vi "EPOS2N~1.VI"() -> ()   [LabVIEW 2017]
doc: "Example of controlling 1 EPOS2 drive in current mode."
uses:
  <vilib>/addons/Maxon Motor/EPOS2 CANopen/EPOS2 Support Files/Typedefs/EPOS2 Status Word PVM.ctl
  <vilib>/addons/Maxon Motor/EPOS2 CANopen/EPOS2 Support Files/Typedefs/EPOS2 Data Output Current.ctl
  <vilib>/addons/Maxon Motor/EPOS2 CANopen/EPOS2 Support Files/Typedefs/EPOS2 Control Word PVM.ctl
  <vilib>/addons/Maxon Motor/EPOS2 CANopen/EPOS2 Support Files/Typedefs/EPOS2 Config Data Input Current.ctl
  <vilib>/addons/Maxon Motor/EPOS2 CANopen/EPOS2 Support Files/Typedefs/EPOS2 Velocity Units.ctl
  <vilib>/Platform/TimedLoop/XDataNode/timing_clust.ctl
  <vilib>/Platform/TimedLoop/XDataNode/nitl_modes.ctl
  <vilib>/Platform/TimedLoop/XDataNode/wakeup.ctl
  <vilib>/addons/Maxon Motor/EPOS2 CANopen/EPOS2 Support Files/Polymorphic SubVIs/Config/EPOS2 Current Mode Configure.vi
  <vilib>/addons/Maxon Motor/EPOS2 CANopen/EPOS2 Support Files/Polymorphic SubVIs/Write PDO/EPOS2 Current Mode Write.vi
  <vilib>/addons/Maxon Motor/EPOS2 CANopen/EPOS2 Support Files/Polymorphic SubVIs/Read PDO/EPOS2 Current Mode Read.vi
  <vilib>/addons/Maxon Motor/EPOS2 CANopen/CANopen/sbCANopenBaseClass.lvclass
  <vilib>/Platform/TimedLoop/XDataNode/XDataNode.xnode
  <vilib>/Platform/TimedLoop/XDataNode/XDNodeRunTimeDep.lvlib
  <vilib>/addons/Maxon Motor/EPOS2 CANopen/EPOS2 Library.lvlib
  <vilib>/addons/Maxon Motor/EPOS2 CANopen/CANopen/CANopen IndCom Interface/sdCANopenIndCom.lvclass
panel:
  in  "Node ID 2":u8=1
  out "error out 2":errorcluster
  in  "stop 2":bool
  out "Status 2":T1
  in  "Current 2":i32(slide) scale=-1000.0..1000.0
  in  "Enable 2":bool
  out "Data Output 2":T2
  out "Data Output":T2
  in  "Enable":bool
  in  "Current":i32(slide) scale=-1000.0..1000.0
  in  "Node ID":u8=1
  out "error out":errorcluster
  out "Status":T1
  in  "stop":bool
  # "This Example VI demonstrates how to control the current of an EPOS2 drive using a CANopen interface.\n\nThis VI must be run from a LabVIEW Project. An Example Projects can be found at: \nC:\\Program Files\\National Instruments\\LabVIEW 2015\\examples\\Maxon Motor\\Maxon EPOS2\nor simliar relative path to current LabVIEW version install location for all opperating systems"
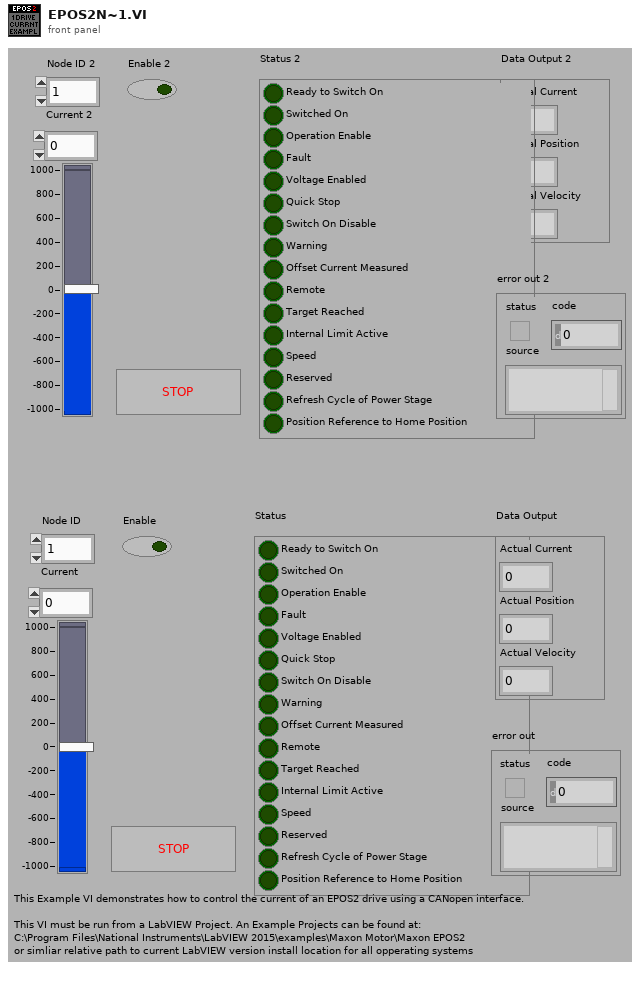
[diagram p1: front panel]
types:
  T1 = typedef "EPOS2 Library.lvlib/EPOS2 Status Word PVM.ctl" = cluster{"Ready to Switch On":bool, "Switched On":bool, "Operation Enable":bool, "Fault":bool, "Voltage Enabled":bool, "Quick Stop":bool, "Switch On Disable":bool, "Warning":bool, "Offset Current Measured":bool, "Remote":bool, "Target Reached":bool, "Internal Limit Active":bool, "Speed":bool, "Reserved":bool, "Refresh Cycle of Power Stage":bool, "Position Reference to Home Position":bool}
  T2 = typedef "EPOS2 Library.lvlib/EPOS2 Data Output Current.ctl" = cluster{"Actual Current":i16, "Actual Position":i32, "Actual Velocity":i32}
  T3 = typedef "EPOS2 Library.lvlib/EPOS2 Config Data Input Current.ctl" = cluster{"Velocity Units":T4, "Max Velocity":i32}
  T4 = typedef "EPOS2 Library.lvlib/EPOS2 Velocity Units.ctl" = i8
  T5 = typedef "EPOS2 Library.lvlib/EPOS2 Control Word PVM.ctl" = cluster{"Switch On":bool, "Enable Voltage":bool, "Quick Stop":bool, "Enable Operation":bool, "Reserved 0":bool, "Reserved 1":bool, "Reserved 2":bool, "Fault Reset":bool, "Halt":bool}
  T6 = typedef "XDNodeRunTimeDep.lvlib/timing_clust.ctl" = cluster{"Expected End [f-1]":u64, "Actual End [f-1]":u64, "Finished Late? [f-1]":bool, "Expected End [i-1]":u64, "Actual End [i-1]":u64, "Finished Late? [i-1]":bool, "Expected Start [i]":u64, "Actual Start [i]":u64, "Expected Start [f]":u64, "Actual Start [f]":u64, "Source Name":string, "Structure Name":string, "Period":i64, "Deadline":i64, "Offset":i64, "Start":i64, "Priority":i32, "Timeout":i32, "Mode":T7, "Wakeup Reason":T8, "Error":errorcluster, "Source Type":string, "Secondary Source Type":string, "Global End Time":u64, "Global Start Time":u64, "Frame Duration":u64, "Iteration Duration":u64, "Assigned CPU":i32, "I/O Scan Engine Mode":u32}
  T7 = typedef "XDNodeRunTimeDep.lvlib/nitl_modes.ctl" = enum32{"No Change", "Process missed periods, maintain original phase", "Discard missed periods, maintain original phase", "Process missed periods, ignore original phase", "Discard missed periods, ignore original phase"}
  T8 = typedef "XDNodeRunTimeDep.lvlib/wakeup.ctl" = enum32{"Normal", "Aborted", "Asynchronous wakeup", "Timing source error", "Timed loop error", "Timeout"}
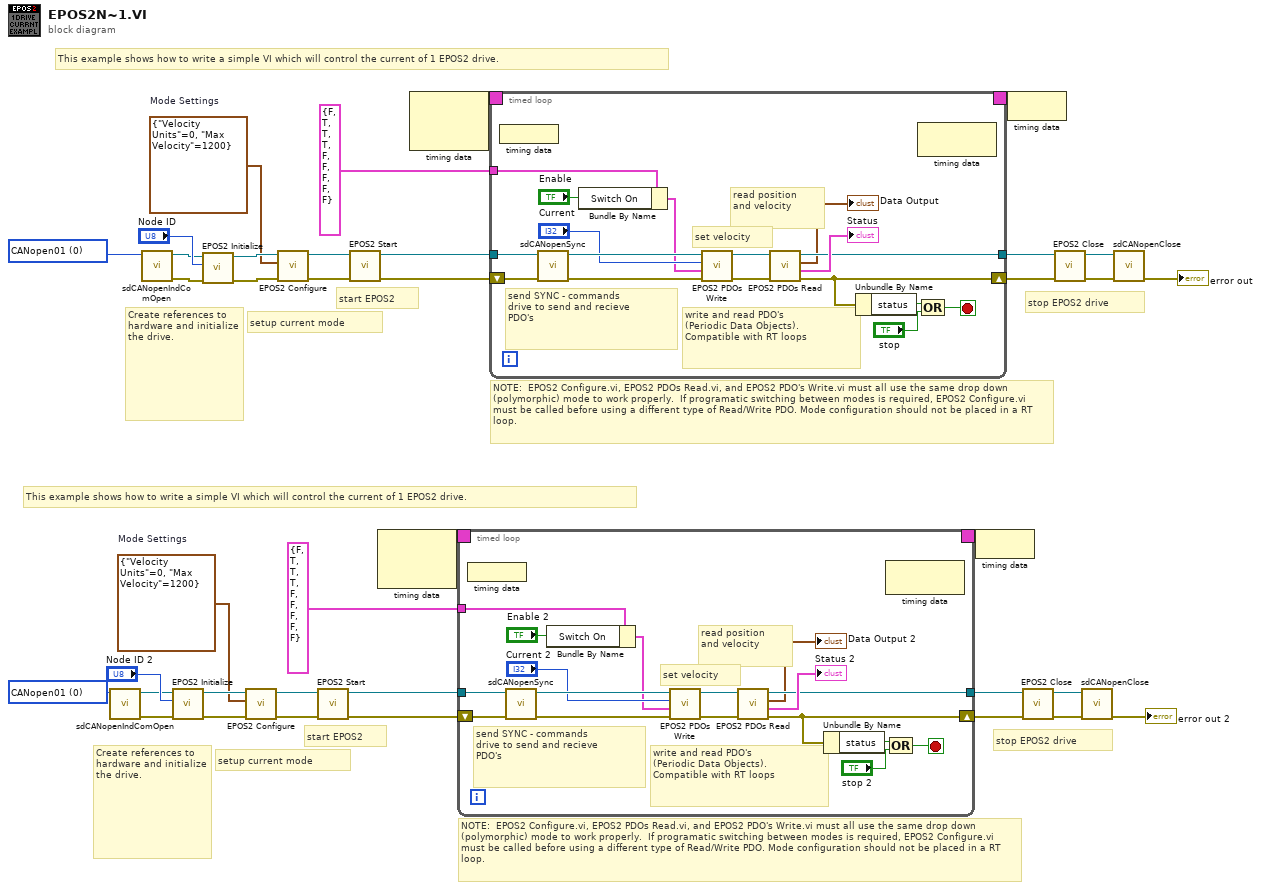
[diagram p0: block diagram]
diagram:
  w2 = u32 0 items=["CANopen01", "CANopen02", "CANopen03", "CANopen04", "CANopen05", "CANopen06", "CANopen07", "CANopen08", "CANopen09", "CANopen10", "CANopen11", "CANopen12", "CANopen13", "CANopen14", "CANopen15", "CANopen16", "CANopen17", "CANopen18", "CANopen19", "CANopen20", "CANopen21", "CANopen22", "CANopen23", "CANopen24", "CANopen25", "CANopen26", "CANopen27", "CANopen28", "CANopen29", "CANopen30", "CANopen31", "CANopen32"] ("Interface Name")
  w7 = T3 {"Velocity Units"=0, "Max Velocity"=1200}  # Mode Settings
  w21 = u32 0 items=["CANopen01", "CANopen02", "CANopen03", "CANopen04", "CANopen05", "CANopen06", "CANopen07", "CANopen08", "CANopen09", "CANopen10", "CANopen11", "CANopen12", "CANopen13", "CANopen14", "CANopen15", "CANopen16", "CANopen17", "CANopen18", "CANopen19", "CANopen20", "CANopen21", "CANopen22", "CANopen23", "CANopen24", "CANopen25", "CANopen26", "CANopen27", "CANopen28", "CANopen29", "CANopen30", "CANopen31", "CANopen32"] ("Interface Name")
  w26 = T3 {"Velocity Units"=0, "Max Velocity"=1200}  # Mode Settings
  # "Create references to hardware and initialize the drive."
  # "This example shows how to write a simple VI which will control the current of 1 EPOS2 drive."
  # "stop EPOS2 drive"
  # "start EPOS2"
  # "setup current mode"
  # "NOTE:  EPOS2 Configure.vi, EPOS2 PDOs Read.vi, and EPOS2 PDO's Write.vi must all use the same drop down (polymorphic) mode to work properly.  If programatic switching between modes is required, EPOS2 Configure.vi must be called before using a different type of Read/Write PDO. Mode configuration should not be placed in a RT loop."
  # "Create references to hardware and initialize the drive."
  # "This example shows how to write a simple VI which will control the current of 1 EPOS2 drive."
  # "stop EPOS2 drive"
  # "start EPOS2"
  # "setup current mode"
  # "NOTE:  EPOS2 Configure.vi, EPOS2 PDOs Read.vi, and EPOS2 PDO's Write.vi must all use the same drop down (polymorphic) mode to work properly.  If programatic switching between modes is required, EPOS2 Configure.vi must be called before using a different type of Read/Write PDO. Mode configuration should not be placed in a RT loop."
  n1 = call <vilib>:"sdCANopenIndComOpen.vi"("Interface Name"=w2) -> ("error out"=w14:errorcluster, "SD CANopen Comm out"=w5:refnum<class "sbCANopenBaseClass.lvclass">)  [unwired: 9 in]
  n2 = call <vilib>:"sdCANopenIndComOpen.vi"("Interface Name"=w21) -> ("error out"=w33:errorcluster, "SD CANopen Comm out"=w24:refnum<class "sbCANopenBaseClass.lvclass">)  [unwired: 9 in]
  n3 = call <vilib>:"EPOS2 Initialize.vi"("error in"=w14, "Node ID"="Node ID 2", "CAN Session In"=w5) -> ("error out"=w15:errorcluster, "CANopen Session Out"=w12:refnum<class "sbCANopenBaseClass.lvclass">)  [unwired: 1 in, 6 out]
  n4 = call <vilib>:"EPOS2 Initialize.vi"("error in"=w33, "Node ID"="Node ID", "CAN Session In"=w24) -> ("error out"=w34:errorcluster, "CANopen Session Out"=w31:refnum<class "sbCANopenBaseClass.lvclass">)  [unwired: 1 in, 6 out]
  n5 = call-poly <vilib>:"EPOS2 Configure.vi"("error in"=w15, "Mode Settings"=w7, "CANopen Session In"=w12) -> ("error out"=w13:errorcluster, "CANopen Session Out"=w11:refnum<class "sbCANopenBaseClass.lvclass">)  [unwired: 7 in]
  n6 = call-poly <vilib>:"EPOS2 Configure.vi"("error in"=w34, "Mode Settings"=w26, "CANopen Session In"=w31) -> ("error out"=w32:errorcluster, "CANopen Session Out"=w30:refnum<class "sbCANopenBaseClass.lvclass">)  [unwired: 7 in]
  n7 = call <vilib>:"EPOS2 Start.vi"("error in"=w13, "CANopen Session In"=w11) -> ("error out"=w16:errorcluster, "CANopen Session Out"=w17:refnum<class "sbCANopenBaseClass.lvclass">)  [unwired: 8 in]
  n8 = call <vilib>:"EPOS2 Start.vi"("error in"=w32, "CANopen Session In"=w30) -> ("error out"=w35:errorcluster, "CANopen Session Out"=w36:refnum<class "sbCANopenBaseClass.lvclass">)  [unwired: 8 in]
  n9 = node-c288() -> (w19:T6)  [unwired: 2 out]
  n10 = node-c288() -> (w38:T6)  [unwired: 2 out]
  n11 = timed-loop {
    timing: w19 -> [_]
    timing-out: [_] -> w18
    tunnel: [w46] -> w10
    tunnel: w17 -> [w40]
    shift-right: [w50] -> w9
    shift-left: w16 -> [w53]
    tunnel: T5 {"Switch On"=FALSE, "Enable Voltage"=TRUE, "Quick Stop"=TRUE, "Enable Operation"=TRUE, "Reserved 0"=FALSE, "Reserved 1"=FALSE, "Reserved 2"=FALSE, "Fault Reset"=FALSE, "Halt"=FALSE} ("Control Word") -> [w44]
    stop <- w39 stop-if-true
    # "read position\nand velocity"
    # "set velocity"
    # "write and read PDO's\n(Periodic Data Objects).\nCompatible with RT loops"
    # "send SYNC - commands\ndrive to send and recieve\nPDO's"
    n12 = node-c288() -> ()  [unwired: 1 out]
    n13 = call-dynamic "sdCANopenSync.vi"("error in (no error)"=w53, "sbCANopenBaseClass in"=w40) -> ("error out"=w52:errorcluster, "sbCANopenBaseClass out"=w47:refnum<class "sbCANopenBaseClass.lvclass">)  [unwired: 8 in]
    n14 = Bundle By Name(cluster=w44, "Switch On"="Enable 2") -> (w42:T5)
    n15 = call-poly <vilib>:"EPOS2 PDOs Write.vi"("error in"=w52, "Control Word"=w42, "Current"="Current 2", "CANopen Session In"=w47) -> ("error out"=w51:errorcluster, "CANopen Session Out"=w48:refnum<class "sbCANopenBaseClass.lvclass">)  [unwired: 6 in]
    n16 = call-poly <vilib>:"EPOS2 PDOs Read.vi"("error in"=w51, "CANopen Session In"=w48) -> ("error out"=w50:errorcluster, "Statusword"=→"Status 2":T1, "Data Output"=→"Data Output 2":T2, "CANopen Session Out"=w46:refnum<class "sbCANopenBaseClass.lvclass">)  [unwired: 6 in]
    n17 = Unbundle By Name(w50) -> ("status"=w54:bool)
    n18 = node-c288() -> ()  [unwired: 2 out]
    n19 = Compound Arithmetic op=OR(w54, "stop 2") -> (w39:bool)
  }
  n20 = timed-loop {
    timing: w38 -> [_]
    timing-out: [_] -> w37
    tunnel: [w65] -> w29
    tunnel: w36 -> [w59]
    shift-right: [w69] -> w28
    shift-left: w35 -> [w72]
    tunnel: T5 {"Switch On"=FALSE, "Enable Voltage"=TRUE, "Quick Stop"=TRUE, "Enable Operation"=TRUE, "Reserved 0"=FALSE, "Reserved 1"=FALSE, "Reserved 2"=FALSE, "Fault Reset"=FALSE, "Halt"=FALSE} ("Control Word") -> [w63]
    stop <- w58 stop-if-true
    # "read position\nand velocity"
    # "set velocity"
    # "write and read PDO's\n(Periodic Data Objects).\nCompatible with RT loops"
    # "send SYNC - commands\ndrive to send and recieve\nPDO's"
    n21 = node-c288() -> ()  [unwired: 1 out]
    n22 = call-dynamic "sdCANopenSync.vi"("error in (no error)"=w72, "sbCANopenBaseClass in"=w59) -> ("error out"=w71:errorcluster, "sbCANopenBaseClass out"=w66:refnum<class "sbCANopenBaseClass.lvclass">)  [unwired: 8 in]
    n23 = Bundle By Name(cluster=w63, "Switch On"="Enable") -> (w61:T5)
    n24 = call-poly <vilib>:"EPOS2 PDOs Write.vi"("error in"=w71, "Control Word"=w61, "Current"="Current", "CANopen Session In"=w66) -> ("error out"=w70:errorcluster, "CANopen Session Out"=w67:refnum<class "sbCANopenBaseClass.lvclass">)  [unwired: 6 in]
    n25 = call-poly <vilib>:"EPOS2 PDOs Read.vi"("error in"=w70, "CANopen Session In"=w67) -> ("error out"=w69:errorcluster, "Statusword"=→"Status":T1, "Data Output"=→"Data Output":T2, "CANopen Session Out"=w65:refnum<class "sbCANopenBaseClass.lvclass">)  [unwired: 6 in]
    n26 = Unbundle By Name(w69) -> ("status"=w73:bool)
    n27 = node-c288() -> ()  [unwired: 2 out]
    n28 = Compound Arithmetic op=OR(w73, "stop") -> (w58:bool)
  }
  n29 = node-c288(w18) -> ()
  n30 = node-c288(w37) -> ()
  n31 = call <vilib>:"EPOS2 Close.vi"("error in"=w9, "CANopen Session In"=w10) -> ("error out"=w3:errorcluster, "CANopen Session Out"=w4:refnum<class "sbCANopenBaseClass.lvclass">)  [unwired: 2 in, 6 out]
  n32 = call <vilib>:"EPOS2 Close.vi"("error in"=w28, "CANopen Session In"=w29) -> ("error out"=w22:errorcluster, "CANopen Session Out"=w23:refnum<class "sbCANopenBaseClass.lvclass">)  [unwired: 2 in, 6 out]
  n33 = call-dynamic "sdCANopenClose.vi"("error in (no error)"=w3, "sbCANopenBaseClass in"=w4) -> ("error out"=→"error out 2":errorcluster)  [unwired: 8 in, 1 out]
  n34 = call-dynamic "sdCANopenClose.vi"("error in (no error)"=w22, "sbCANopenBaseClass in"=w23) -> ("error out"=→"error out":errorcluster)  [unwired: 8 in, 1 out]
